vi "Configure Jitter Real Time Eye Analysis.vi"(8 "error in (no error)":errorcluster, 9 "Real Time Eye Source (1: Channel 1)":i32(ring)=1 items=["Channel 1"=1, "Channel 2"=2, "Channel 3"=3, "Channel 4"=4], 10 "Enable Real Time Eye Analysis (T: Enable)":bool=TRUE, 11 "VISA resource name":refnum<visa-resource-name>) -> (0 "error out":errorcluster, 3 "VISA resource name out":refnum<visa-resource-name>)   [LabVIEW 2015, in "Agilent 2000 3000 X-Series.lvlib"]
doc: "Enables and configures Real Time Eye Analysis.\n\n<b>Note:</b>\nThis VI is specific to the 6000-X Series oscilloscopes. These features are not available on other models."
uses:
  Agilent 2000 3000 X-Series.lvlib
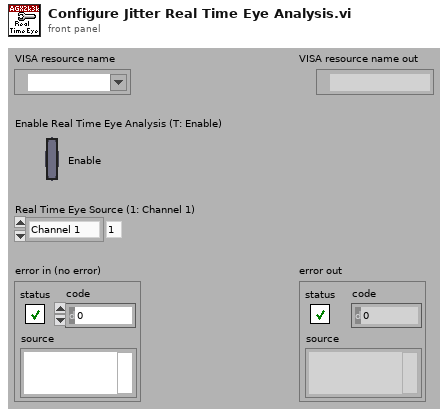
[diagram p1: front panel]
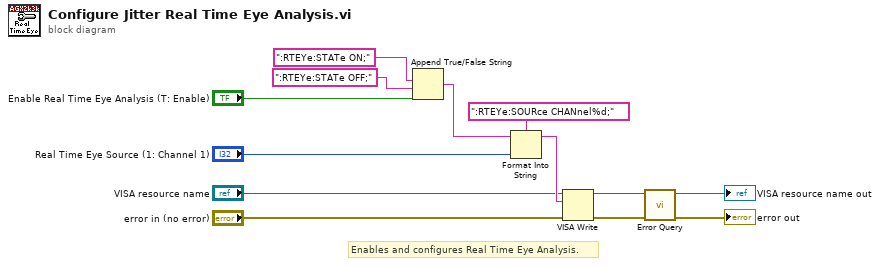
[diagram p0: block diagram]
diagram:
  # "Enables and configures Real Time Eye Analysis."
  n1 = Append True/False String(1:"Enable Real Time Eye Analysis (T: Enable)", 2:":RTEYe:STATe OFF;", 3:":RTEYe:STATe ON;") -> (0:w10:string)  [unwired: 1 in]
  n2 = Format Into String(format string=":RTEYe:SOURce CHANnel%d;", initial string=w10, "Real Time Eye Source (1: Channel 1)") -> (resulting string=w7:string)  [unwired: 1 in, 1 out]
  n3 = VISA Write(VISA resource name="VISA resource name", write buffer=w7, error in (no error)="error in (no error)") -> (VISA resource name out=w4:refnum<visa-resource-name>, error out=w3:errorcluster)  [unwired: 1 out]
  n4 = call "Error Query.vi"("error in (no error)"=w3, "VISA resource name"=w4) -> ("error out"=→"error out":errorcluster, "VISA resource name out"=→"VISA resource name out":refnum<visa-resource-name>)  [unwired: 6 in, 2 out]
